vi "Tosca-Reexecute Script.vi"(0 "State in":refnum<class "State.lvclass">, 2 "Tosca":refnum<class "Parameters.lvclass">, 11 "error in (no error)":errorcluster) -> (4 "State out":refnum<class "State.lvclass">, 15 "error out":errorcluster)   [LabVIEW 2020]
uses:
  Classes/State/State.lvclass
  Classes/Parameters/Parameters.lvclass
  Classes/State/State.lvclass/State.ctl
  Classes/Parameters/Parameters.lvclass/Parameters.ctl
  Classes/Parameters/Read Pretrial.vi
  Classes/Parameters/Read DAQ.vi
  Classes/State/Read script.vi
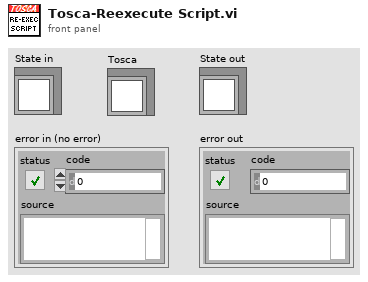
[diagram p1: front panel]
types:
  T1 = typedef "Tosca-Pretrial Spec.ctl" = cluster{"Path":path, "Args":string[]}
  T2 = typedef "Parameters.lvclass/DAQ.ctl" = cluster{"AO Fs (Hz)":dbl, "DO Fs (Hz)":dbl, "Poll Rate (Hz)":dbl, "Baseline (s)":dbl}
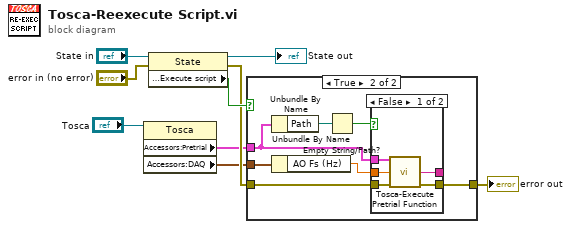
[diagram p0: block diagram]
diagram:
  n1 = property class="Tosca"(reference="Tosca") -> ("Accessors:Pretrial"=w3:T1, "Accessors:DAQ"=w2:T2)  [unwired: 1 in, 2 out]
  n2 = property class="State"(reference="State in", error in="error in (no error)") -> (reference out=→"State out":refnum<class "State.lvclass">, error out=w5:errorcluster, "Accessors:Execute script"=w6:bool)
  n3 = case shown="True" w6 {
    tunnel: w5 -> [w10 w17]
    tunnel: w3 -> [_ w11]
    tunnel: w2 -> [_ w16]
    tunnel: [w10 w12] -> w1
    frame False {
    }
    frame True {
      n4 = Unbundle By Name(w11) -> ("Path"=w13:path)
      n5 = Unbundle By Name(w16) -> ("AO Fs (Hz)"=w15:dbl)
      n6 = Empty String/Path?(string/path=w13) -> (empty?=w14:bool)
      n7 = case shown="False" w14 {
        tunnel: [w22 _] -> w12
        tunnel: w11 -> [w21 _]
        tunnel: w15 -> [w20 _]
        tunnel: [w19 _] -> _
        tunnel: w17 -> [w18 _]
        frame False {
          n8 = call "Tosca-Execute Pretrial Function.vi"("Pretrial in"=w21, "Fs"=w20, "error in (no error)"=w18) -> ("output"=w19:string, "error out"=w22:errorcluster)  [unwired: 11 in]
        }
        frame True {
        }
      }
    }
  }
  "error out" <- w1
